vi "Correlation.vi"(1 "ANN outputs":sgl[](array[numeric]) format="%.2f", 2 "Targets":sgl[](array[numeric]) format="%.2f") -> (0 "Correlation":sgl format="%.2e")   [LabVIEW 2010]
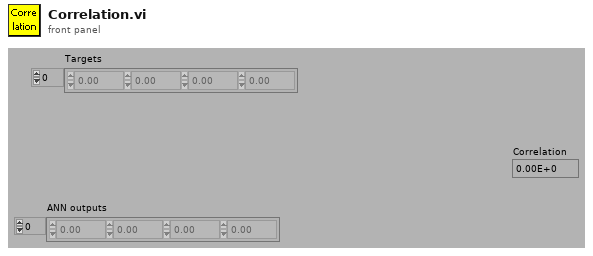
[diagram p1: front panel]
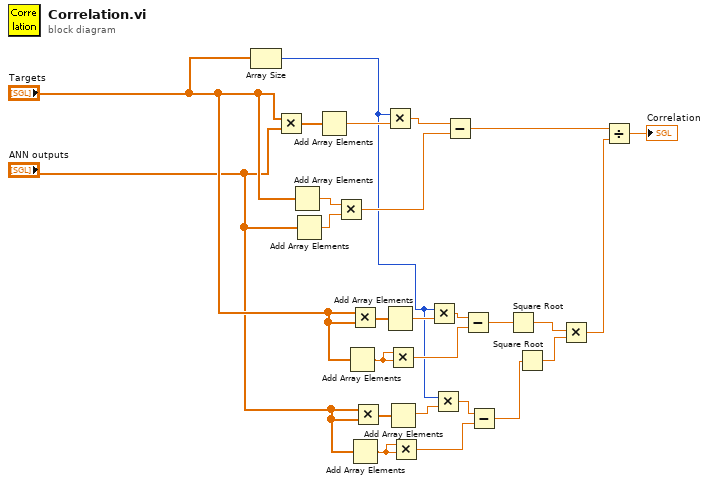
[diagram p0: block diagram]
diagram:
  n1 = Array Size(array="Targets") -> (size(s)=w8:i32)
  n2 = Multiply(x="Targets", y="ANN outputs") -> (x*y=w26:sgl[])
  n3 = Add Array Elements(numeric array="Targets") -> (sum=w24:sgl)
  n4 = Add Array Elements(numeric array="ANN outputs") -> (sum=w23:sgl)
  n5 = Add Array Elements(numeric array=w26) -> (sum=w25:sgl)
  n6 = Multiply(x=w24, y=w23) -> (x*y=w15:sgl)
  n7 = Add Array Elements(numeric array="Targets") -> (sum=w20:sgl)
  n8 = Multiply(x="Targets", y="Targets") -> (x*y=w21:sgl[])
  n9 = Add Array Elements(numeric array="ANN outputs") -> (sum=w19:sgl)
  n10 = Multiply(x="ANN outputs", y="ANN outputs") -> (x*y=w18:sgl[])
  n11 = Multiply(x=w8, y=w25) -> (x*y=w16:sgl)
  n12 = Add Array Elements(numeric array=w21) -> (sum=w13:sgl)
  n13 = Multiply(x=w20, y=w20) -> (x*y=w14:sgl)
  n14 = Add Array Elements(numeric array=w18) -> (sum=w7:sgl)
  n15 = Multiply(x=w19, y=w19) -> (x*y=w5:sgl)
  n16 = Multiply(x=w8, y=w13) -> (x*y=w12:sgl)
  n17 = Multiply(x=w8, y=w7) -> (x*y=w6:sgl)
  n18 = Subtract(x=w16, y=w15) -> (x-y=w22:sgl)
  n19 = Subtract(x=w12, y=w14) -> (x-y=w11:sgl)
  n20 = Subtract(x=w6, y=w5) -> (x-y=w4:sgl)
  n21 = Square Root(x=w11) -> (sqrt(x)=w9:sgl)
  n22 = Square Root(x=w4) -> (sqrt(x)=w3:sgl)
  n23 = Multiply(x=w9, y=w3) -> (x*y=w10:sgl)
  n24 = Divide(x=w22, y=w10) -> (x/y=→"Correlation":sgl)
